vi "get_pck_data.vi"(11 "w5500_pck":T1) -> (3 "Numeric":u32)   [LabVIEW 2021]
uses:
  typedefs/w5500_pck.ctl
  typedefs/w5500_cmd.ctl
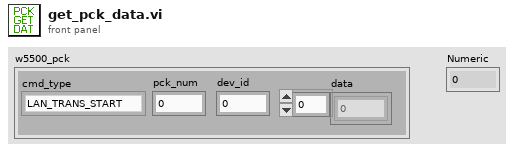
[diagram p1: front panel]
types:
  T1 = typedef "w5500_pck.ctl" = cluster{"cmd_type":T2, "pck_num":u32, "dev_id":u32, "data":u8[]}
  T2 = typedef "w5500_cmd.ctl" = enum32{"LAN_TRANS_START", "LAN_DATA_SZ", "LAN_CHUNK_SEND", "LAN_CHUNK_ACK", "LAN_DEVS_INFO", "LAN_DEVS_NUM", "LAN_DEVS_EXS", "LAN_DEVS_ACK", "LAN_CMD_ACK", "LAN_CMD_FIN", "LAN_SND_STAT", "LAN_REQ_STAT", "LAN_ANS_STAT", "LAN_ERR_STAT", "LAN_SETT_SET", "LAN_SETT_GET", "LAN_SETT_ACK", "LAN_SETT_ERR"}
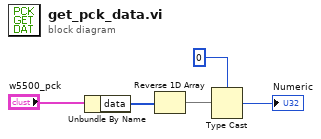
[diagram p0: block diagram]
diagram:
  n1 = Unbundle By Name("w5500_pck") -> ("data"=w3:u8[])
  n2 = Reverse 1D Array(array=w3) -> (reversed array=w4:u8[])
  n3 = Type Cast(type=u32 0, x=w4) -> (*(type *) &x=→"Numeric":u32)
